vi "Lab Panel V5.11.vi"() -> ()   [LabVIEW 2013] (continued)
                        }
                        n855 = Bundle(cluster=w1527, "STATUS"="STOP") -> (w1525:T4)  [unwired: 2 in]
                        n856 = local write "DISP LAB04-1"(w1525) -> ()
                      }
                    }
                  }
                  frame True {
                    n857 = local read "SIG LAB04-1"() -> (w1534:T2)
                    n858 = stacked-sequence {
                      seq-local: [w1545 _] -> [_ w1549]
                      tunnel: w1543 -> [_ w1559]
                      tunnel: w1542 -> [_ w1558]
                      tunnel: w1541 -> [_ w1557]
                      tunnel: w1540 -> [_ w1556]
                      tunnel: w1539 -> [_ w1555]
                      tunnel: [_ w1554] -> w1538
                      tunnel: w1537 -> [_ w1553]
                      tunnel: w1536 -> [_ w1552]
                      tunnel: w1535 -> [_ w1551]
                      tunnel: w1534 -> [w1544 w1550]
                      tunnel: w1533 -> [_ w1548]
                      frame #0 {
                        n859 = Unbundle(w1544) -> ("AMPS"=w1547:dbl)  [unwired: 4 out]
                        n860 = call "Check For Amps on v1.vi"("ID"="LAB04-1", "amps"=w1547) -> ("amps"=w1545:bool)  [unwired: 9 in]
                      }
                      frame #1 {
                        n861 = case shown="True" w1549 {
                          tunnel: w1559 -> [_ w1572]
                          tunnel: w1558 -> [_ w1571]
                          tunnel: w1557 -> [_ w1570]
                          tunnel: w1556 -> [_ w1569]
                          tunnel: w1555 -> [_ w1568]
                          tunnel: [errorcluster {"status"=FALSE, "code"=0, "source"=""} ("error out") w1567] -> w1554
                          tunnel: w1553 -> [_ w1566]
                          tunnel: w1552 -> [_ w1565]
                          tunnel: w1551 -> [_ w1564]
                          tunnel: w1550 -> [_ w1563]
                          tunnel: w1548 -> [_ w1562]
                          frame False {
                            w1560 = FALSE
                            n862 = local write "RUN LAB04-1"(w1560) -> ()
                            n863 = local write "run lab04-1"(w1560) -> ()
                          }
                          frame True {
                            n864 = stacked-sequence {
                              seq-local: [w1573 _ _ _ _] -> [_ w1597 _ _ _]
                              tunnel: w1572 -> [w1578 _ _ _ _]
                              tunnel: w1571 -> [w1574 _ _ _ _]
                              tunnel: w1570 -> [w1588 _ _ _ _]
                              tunnel: w1569 -> [w1581 _ _ _ _]
                              tunnel: w1568 -> [w1576 _ _ _ _]
                              tunnel: [_ w1592 _ _ _] -> w1567
                              tunnel: w1566 -> [_ _ _ w1618 _]
                              tunnel: w1565 -> [_ _ _ w1617 _]
                              tunnel: w1564 -> [_ _ _ w1616 _]
                              tunnel: w1563 -> [_ _ _ _ _]
                              tunnel: w1562 -> [_ _ _ _ w1632]
                              frame #0 {
                                w1575 = "\\"
                                n865 = local read "SET LAB04-1"() -> (w1583:T5)
                                n866 = case shown="\"CYCLE TEST\"" w1588 {
                                tunnel: ["L04-1-CHART TEST-" "L04-1-CYCLE TEST-" "L04-1-T-RISE TEST-"] -> w1584
                                frame "CHART TEST", Default {
                                }
                                frame "CYCLE TEST" {
                                }
                                frame "T-RISE TEST" {
                                }
                                }
                                n867 = Unbundle(w1583) -> ("DESCRIPTION"=w1582:string)  [unwired: 4 out]
                                n868 = Concatenate Strings(w1578, "\\", w1576, w1575, w1574, w1575) -> (w1585:string)
                                n869 = String To Path(string=w1585) -> (path=w1587:path)
                                n870 = Concatenate Strings(w1585, w1584, w1582, "-", w1581, ".tdms") -> (w1573:string)
                                n871 = Create Folder(path (use dialog)=w1587) -> (error out=w1586:errorcluster)  [unwired: 2 in, 2 out]
                                n872 = global write "Global 1.vi" "LAB04-1 FILE"(w1573) -> ()
                                n873 = call <vilib>:"Clear Errors.vi"("error in (no error)"=w1586) -> ()  [unwired: 6 in, 1 out]
                              }
                              frame #1 {
                                (unwired) FALSE
                                n874 = String To Path(string=w1597) -> (path=w1593:path)
                                n875 = TDMS Open(6:FALSE, 10:T20."create or replace" ("operation (0:open)"), 11:w1593) -> (0:w1592:errorcluster, 3:→"TDMS LAB04-1":refnum<k34>)  [unwired: 4 in]
                              }
                              frame #2 {
                                n876 = local read "SET LAB04-1"() -> (w1603:T5)
                                n877 = local read "TDMS LAB04-1"() -> (w1614:refnum<k34>)
                                n878 = Build Array("Testers Name", "Description", "Set Test Cycles", "T-Rise minutes", "T-Rise Deg C") -> (w1604:string[])
                                n879 = Unbundle(w1603) -> ("NAME"=w1602:string, "DESCRIPTION"=w1601:string, "CYCLES"=w1600:dbl, "T-RISE mins"=w1599:dbl, "T-RISE deg C"=w1598:dbl)
                                n880 = Number To Decimal String(number=w1600) -> (decimal integer string=w1613:string)  [unwired: 1 in]
                                n881 = Number To Decimal String(number=w1599) -> (decimal integer string=w1612:string)  [unwired: 1 in]
                                n882 = Number To Decimal String(number=w1598) -> (decimal integer string=w1611:string)  [unwired: 1 in]
                                n883 = Build Array(w1602, w1601, w1613, w1612, w1611) -> (w1610:string[])
                                n884 = TDMS Set Properties(5:w1610, 7:w1604, 11:w1614) -> ()  [unwired: 3 in, 4 out]
                              }
                              frame #3 {
                                n885 = local read "DISP LAB04-1"() -> (w1619:T4)
                                n886 = Concatenate Strings("LAB04-1  ", w1618) -> (w1620:string)
                                n887 = Two Button Dialog(message=w1620, 1:w1616, 2:w1617) -> (T button?=w1622:bool)
                                n888 = case shown="True" w1622 {
                                tunnel: w1619 -> [w1629 w1630]
                                tunnel: [w1629 w1630] -> w1626
                                tunnel: [w1628 w1631] -> w1625
                                tunnel: [w1627 w1631] -> w1624
                                frame False {
                                n889 = Unbundle(w1629) -> ("CYCLE"=w1628:dbl, "MINS"=w1627:dbl)  [unwired: 1 out]
                                }
                                frame True {
                                w1631 = 0.0
                                }
                                }
                                n890 = Bundle(cluster=w1626, "CYCLE"=w1625, "MINS"=w1624, "STATUS"="RUN") -> (w1615:T4)
                                n891 = local write "DISP LAB04-1"(w1615) -> ()
                              }
                              frame #4 {
                                n892 = local read "TEMP START LAB04-1"() -> (w1634:cluster{"TL":dbl, "TN":dbl})
                                n893 = Bundle(cluster=w1634, "TL"=w1632, "TN"=w1632) -> (w1633:cluster{"TL":dbl, "TN":dbl})
                                n894 = local write "TEMP START LAB04-1"(w1633) -> ()
                              }
                            }
                          }
                        }
                      }
                    }
                  }
                }
              }
              event "RUN LAB04-2": Value Change {
                n895 = event-data() -> ("NewVal"=w1639:bool)  [unwired: 1 in, 5 out]
                n896 = local write "run lab04-2"(w1639) -> ()
                n897 = case shown="True" w1639 {
                  tunnel: w1645 -> [_ w1683]
                  tunnel: w1644 -> [_ w1682]
                  tunnel: w1642 -> [w1647 w1681]
                  tunnel: w1643 -> [_ w1680]
                  tunnel: w1641 -> [_ w1679]
                  tunnel: [w1646 w1678] -> w1640
                  tunnel: w1638 -> [_ w1677]
                  tunnel: w1637 -> [_ w1676]
                  tunnel: w1636 -> [_ w1675]
                  tunnel: w1635 -> [_ w1673]
                  frame False {
                    # "stop test"
                    n898 = stacked-sequence {
                      tunnel: w1647 -> [w1656 _]
                      tunnel: [w1648 _] -> w1646
                      frame #0 {
                        n899 = local read "DISP LAB04-2"() -> (w1655:T4)
                        n900 = Unbundle(w1655) -> ("CYCLE"=w1653:dbl, "MINS"=w1654:dbl)  [unwired: 1 out]
                        n901 = case shown="\"CYCLE TEST\"" w1656 {
                          tunnel: w1654 -> [_ _ w1663]
                          tunnel: w1653 -> [w1661 w1662 _]
                          tunnel: [w1661 w1662 w1663] -> w1652
                          frame "CHART TEST", Default {
                          }
                          frame "CYCLE TEST" {
                          }
                          frame "T-RISE TEST" {
                          }
                        }
                        n902 = local read "TDMS LAB04-2"() -> (w1660:refnum<k34>)
                        n903 = Build Array("STOPPED") -> (w1657:string[])
                        n904 = Build Array(w1652) -> (w1651:dbl[])
                        n905 = TDMS Write(0:w1660, 5:"TEST RESULT", 7:w1657, 9:w1651) -> (4:w1649:refnum<k34>, 15:w1650:errorcluster)  [unwired: 2 in, 2 out]
                        n906 = TDMS Close(8:w1650, 11:w1649) -> (0:w1648:errorcluster)  [unwired: 1 out]
                      }
                      frame #1 {
                        n907 = local read "DISP LAB04-2"() -> (w1667:T4)
                        n908 = stacked-sequence {
                          tunnel: "LAB04-2" -> [w1669 w1671]
                          frame #0 {
                            n909 = call "sub vi - defrag tdms v1.vi"("panel id"=w1669) -> ("error out"=w1668:errorcluster)  [unwired: 10 in]
                            n910 = local write "data file error"(w1668) -> ()
                          }
                          frame #1 {
                            n911 = call "Save data file (stop) v3.vi"("panel id"=w1671) -> ("network file save error"=w1670:errorcluster)  [unwired: 9 in, 1 out]
                            n912 = local write "RESULT LAB04-2"(FALSE) -> ()
                            n913 = local write "data file error"(w1670) -> ()
                          }
                        }
                        n914 = Bundle(cluster=w1667, "STATUS"="STOP") -> (w1665:T4)  [unwired: 2 in]
                        n915 = local write "DISP LAB04-2"(w1665) -> ()
                      }
                    }
                  }
                  frame True {
                    n916 = local read "SIG LAB04-2"() -> (w1674:T2)
                    n917 = stacked-sequence {
                      seq-local: [w1685 _] -> [_ w1689]
                      tunnel: w1683 -> [_ w1699]
                      tunnel: w1682 -> [_ w1698]
                      tunnel: w1681 -> [_ w1697]
                      tunnel: w1680 -> [_ w1696]
                      tunnel: w1679 -> [_ w1695]
                      tunnel: [_ w1694] -> w1678
                      tunnel: w1677 -> [_ w1693]
                      tunnel: w1676 -> [_ w1692]
                      tunnel: w1675 -> [_ w1691]
                      tunnel: w1674 -> [w1684 w1690]
                      tunnel: w1673 -> [_ w1688]
                      frame #0 {
                        n918 = Unbundle(w1684) -> ("AMPS"=w1687:dbl)  [unwired: 4 out]
                        n919 = call "Check For Amps on v1.vi"("ID"="LAB04-2", "amps"=w1687) -> ("amps"=w1685:bool)  [unwired: 9 in]
                      }
                      frame #1 {
                        n920 = case shown="True" w1689 {
                          tunnel: w1699 -> [_ w1712]
                          tunnel: w1698 -> [_ w1711]
                          tunnel: w1697 -> [_ w1710]
                          tunnel: w1696 -> [_ w1709]
                          tunnel: w1695 -> [_ w1708]
                          tunnel: [errorcluster {"status"=FALSE, "code"=0, "source"=""} ("error out") w1707] -> w1694
                          tunnel: w1693 -> [_ w1706]
                          tunnel: w1692 -> [_ w1705]
                          tunnel: w1691 -> [_ w1704]
                          tunnel: w1690 -> [_ w1703]
                          tunnel: w1688 -> [_ w1702]
                          frame False {
                            w1700 = FALSE
                            n921 = local write "RUN LAB04-2"(w1700) -> ()
                            n922 = local write "run lab04-2"(w1700) -> ()
                          }
                          frame True {
                            n923 = stacked-sequence {
                              seq-local: [w1713 _ _ _ _] -> [_ w1737 _ _ _]
                              tunnel: w1712 -> [w1718 _ _ _ _]
                              tunnel: w1711 -> [w1714 _ _ _ _]
                              tunnel: w1710 -> [w1728 _ _ _ _]
                              tunnel: w1709 -> [w1721 _ _ _ _]
                              tunnel: w1708 -> [w1716 _ _ _ _]
                              tunnel: [_ w1732 _ _ _] -> w1707
                              tunnel: w1706 -> [_ _ _ w1758 _]
                              tunnel: w1705 -> [_ _ _ w1757 _]
                              tunnel: w1704 -> [_ _ _ w1756 _]
                              tunnel: w1703 -> [_ _ _ _ _]
                              tunnel: w1702 -> [_ _ _ _ w1772]
                              frame #0 {
                                w1715 = "\\"
                                n924 = local read "SET LAB04-2"() -> (w1723:T5)
                                n925 = case shown="\"CHART TEST\", Default" w1728 {
                                tunnel: ["L04-2-CHART TEST-" "L04-2-CYCLE TEST-" "L04-2-T-RISE TEST-"] -> w1724
                                frame "CHART TEST", Default {
                                }
                                frame "CYCLE TEST" {
                                }
                                frame "T-RISE TEST" {
                                }
                                }
                                n926 = Unbundle(w1723) -> ("DESCRIPTION"=w1722:string)  [unwired: 4 out]
                                n927 = Concatenate Strings(w1718, "\\", w1716, w1715, w1714, w1715) -> (w1725:string)
                                n928 = String To Path(string=w1725) -> (path=w1727:path)
                                n929 = Concatenate Strings(w1725, w1724, w1722, "-", w1721, ".tdms") -> (w1713:string)
                                n930 = Create Folder(path (use dialog)=w1727) -> (error out=w1726:errorcluster)  [unwired: 2 in, 2 out]
                                n931 = global write "Global 1.vi" "LAB04-2 FILE"(w1713) -> ()
                                n932 = call <vilib>:"Clear Errors.vi"("error in (no error)"=w1726) -> ()  [unwired: 6 in, 1 out]
                              }
                              frame #1 {
                                (unwired) FALSE
                                n933 = String To Path(string=w1737) -> (path=w1733:path)
                                n934 = TDMS Open(6:FALSE, 10:T20."create or replace" ("operation (0:open)"), 11:w1733) -> (0:w1732:errorcluster, 3:→"TDMS LAB04-2":refnum<k34>)  [unwired: 4 in]
                              }
                              frame #2 {
                                n935 = local read "SET LAB04-2"() -> (w1743:T5)
                                n936 = local read "TDMS LAB04-2"() -> (w1754:refnum<k34>)
                                n937 = Build Array("Testers Name", "Description", "Set Test Cycles", "T-Rise minutes", "T-Rise Deg C") -> (w1744:string[])
                                n938 = Unbundle(w1743) -> ("NAME"=w1742:string, "DESCRIPTION"=w1741:string, "CYCLES"=w1740:dbl, "T-RISE mins"=w1739:dbl, "T-RISE deg C"=w1738:dbl)
                                n939 = Number To Decimal String(number=w1740) -> (decimal integer string=w1753:string)  [unwired: 1 in]
                                n940 = Number To Decimal String(number=w1739) -> (decimal integer string=w1752:string)  [unwired: 1 in]
                                n941 = Number To Decimal String(number=w1738) -> (decimal integer string=w1751:string)  [unwired: 1 in]
                                n942 = Build Array(w1742, w1741, w1753, w1752, w1751) -> (w1750:string[])
                                n943 = TDMS Set Properties(5:w1750, 7:w1744, 11:w1754) -> ()  [unwired: 3 in, 4 out]
                              }
                              frame #3 {
                                n944 = local read "DISP LAB04-2"() -> (w1759:T4)
                                n945 = Concatenate Strings("LAB04-2 ", w1758) -> (w1760:string)
                                n946 = Two Button Dialog(message=w1760, 1:w1756, 2:w1757) -> (T button?=w1762:bool)
                                n947 = case shown="True" w1762 {
                                tunnel: w1759 -> [w1769 w1770]
                                tunnel: [w1769 w1770] -> w1766
                                tunnel: [w1768 w1771] -> w1765
                                tunnel: [w1767 w1771] -> w1764
                                frame False {
                                n948 = Unbundle(w1769) -> ("CYCLE"=w1768:dbl, "MINS"=w1767:dbl)  [unwired: 1 out]
                                }
                                frame True {
                                w1771 = 0.0
                                }
                                }
                                n949 = Bundle(cluster=w1766, "CYCLE"=w1765, "MINS"=w1764, "STATUS"="RUN") -> (w1755:T4)
                                n950 = local write "DISP LAB04-2"(w1755) -> ()
                              }
                              frame #4 {
                                n951 = local read "TEMP START LAB04-2"() -> (w1774:cluster{"TL":dbl, "TN":dbl})
                                n952 = Bundle(cluster=w1774, "TL"=w1772, "TN"=w1772) -> (w1773:cluster{"TL":dbl, "TN":dbl})
                                n953 = local write "TEMP START LAB04-2"(w1773) -> ()
                              }
                            }
                          }
                        }
                      }
                    }
                  }
                }
              }
              event "RUN LAB05-1": Value Change {
                n954 = event-data() -> ("NewVal"=w1779:bool)  [unwired: 1 in, 5 out]
                n955 = local write "run lab05-1"(w1779) -> ()
                n956 = case shown="True" w1779 {
                  tunnel: w1785 -> [_ w1823]
                  tunnel: w1784 -> [_ w1822]
                  tunnel: w1782 -> [w1787 w1821]
                  tunnel: w1783 -> [_ w1820]
                  tunnel: w1781 -> [_ w1819]
                  tunnel: [w1786 w1818] -> w1780
                  tunnel: w1778 -> [_ w1817]
                  tunnel: w1777 -> [_ w1816]
                  tunnel: w1776 -> [_ w1815]
                  tunnel: w1775 -> [_ w1813]
                  frame False {
                    # "stop test"
                    n957 = stacked-sequence {
                      tunnel: w1787 -> [w1796 _]
                      tunnel: [w1788 _] -> w1786
                      frame #0 {
                        n958 = local read "DISP LAB05-1"() -> (w1795:T4)
                        n959 = Unbundle(w1795) -> ("CYCLE"=w1793:dbl, "MINS"=w1794:dbl)  [unwired: 1 out]
                        n960 = case shown="\"CYCLE TEST\"" w1796 {
                          tunnel: w1794 -> [_ _ w1803]
                          tunnel: w1793 -> [w1801 w1802 _]
                          tunnel: [w1801 w1802 w1803] -> w1792
                          frame "CHART TEST", Default {
                          }
                          frame "CYCLE TEST" {
                          }
                          frame "T-RISE TEST" {
                          }
                        }
                        n961 = local read "TDMS LAB05-1"() -> (w1800:refnum<k34>)
                        n962 = Build Array("STOPPED") -> (w1797:string[])
                        n963 = Build Array(w1792) -> (w1791:dbl[])
                        n964 = TDMS Write(0:w1800, 5:"TEST RESULT", 7:w1797, 9:w1791) -> (4:w1789:refnum<k34>, 15:w1790:errorcluster)  [unwired: 2 in, 2 out]
                        n965 = TDMS Close(8:w1790, 11:w1789) -> (0:w1788:errorcluster)  [unwired: 1 out]
                      }
                      frame #1 {
                        n966 = local read "DISP LAB05-1"() -> (w1807:T4)
                        n967 = stacked-sequence {
                          tunnel: "LAB05-1" -> [w1809 w1811]
                          frame #0 {
                            n968 = call "sub vi - defrag tdms v1.vi"("panel id"=w1809) -> ("error out"=w1808:errorcluster)  [unwired: 10 in]
                            n969 = local write "data file error"(w1808) -> ()
                          }
                          frame #1 {
                            n970 = call "Save data file (stop) v3.vi"("panel id"=w1811) -> ("network file save error"=w1810:errorcluster)  [unwired: 9 in, 1 out]
                            n971 = local write "RESULT LAB05-1"(FALSE) -> ()
                            n972 = local write "data file error"(w1810) -> ()
                          }
                        }
                        n973 = Bundle(cluster=w1807, "STATUS"="STOP") -> (w1805:T4)  [unwired: 2 in]
                        n974 = local write "DISP LAB05-1"(w1805) -> ()
                      }
                    }
                  }
                  frame True {
                    n975 = local read "SIG LAB05-1"() -> (w1814:T2)
                    n976 = stacked-sequence {
                      seq-local: [w1825 _] -> [_ w1829]
                      tunnel: w1823 -> [_ w1839]
                      tunnel: w1822 -> [_ w1838]
                      tunnel: w1821 -> [_ w1837]
                      tunnel: w1820 -> [_ w1836]
                      tunnel: w1819 -> [_ w1835]
                      tunnel: [_ w1834] -> w1818
                      tunnel: w1817 -> [_ w1833]
                      tunnel: w1816 -> [_ w1832]
                      tunnel: w1815 -> [_ w1831]
                      tunnel: w1814 -> [w1824 w1830]
                      tunnel: w1813 -> [_ w1828]
                      frame #0 {
                        n977 = Unbundle(w1824) -> ("AMPS"=w1827:dbl)  [unwired: 4 out]
                        n978 = call "Check For Amps on v1.vi"("ID"="LAB05-1", "amps"=w1827) -> ("amps"=w1825:bool)  [unwired: 9 in]
                      }
                      frame #1 {
                        n979 = case shown="True" w1829 {
                          tunnel: w1839 -> [_ w1852]
                          tunnel: w1838 -> [_ w1851]
                          tunnel: w1837 -> [_ w1850]
                          tunnel: w1836 -> [_ w1849]
                          tunnel: w1835 -> [_ w1848]
                          tunnel: [errorcluster {"status"=FALSE, "code"=0, "source"=""} ("error out") w1847] -> w1834
                          tunnel: w1833 -> [_ w1846]
                          tunnel: w1832 -> [_ w1845]
                          tunnel: w1831 -> [_ w1844]
                          tunnel: w1830 -> [_ w1843]
                          tunnel: w1828 -> [_ w1842]
                          frame False {
                            w1840 = FALSE
                            n980 = local write "RUN LAB05-1"(w1840) -> ()
                            n981 = local write "run lab05-1"(w1840) -> ()
                          }
                          frame True {
                            n982 = stacked-sequence {
                              seq-local: [w1853 _ _ _ _] -> [_ w1877 _ _ _]
                              tunnel: w1852 -> [w1858 _ _ _ _]
                              tunnel: w1851 -> [w1854 _ _ _ _]
                              tunnel: w1850 -> [w1868 _ _ _ _]
                              tunnel: w1849 -> [w1861 _ _ _ _]
                              tunnel: w1848 -> [w1856 _ _ _ _]
                              tunnel: [_ w1872 _ _ _] -> w1847
                              tunnel: w1846 -> [_ _ _ w1897 _]
                              tunnel: w1845 -> [_ _ _ w1896 _]
                              tunnel: w1844 -> [_ _ _ w1895 _]
                              tunnel: w1843 -> [_ _ _ _ _]
                              tunnel: w1842 -> [_ _ _ _ w1912]
                              frame #0 {
                                w1855 = "\\"
                                n983 = local read "SET LAB05-1"() -> (w1863:T5)
                                n984 = case shown="\"CYCLE TEST\"" w1868 {
                                tunnel: ["L05-1-CHART TEST-" "L05-1-CYCLE TEST-" "L05-1-T-RISE TEST-"] -> w1864
                                frame "CHART TEST", Default {
                                }
                                frame "CYCLE TEST" {
                                }
                                frame "T-RISE TEST" {
                                }
                                }
                                n985 = Unbundle(w1863) -> ("DESCRIPTION"=w1862:string)  [unwired: 4 out]
                                n986 = Concatenate Strings(w1858, "\\", w1856, w1855, w1854, w1855) -> (w1865:string)
                                n987 = String To Path(string=w1865) -> (path=w1867:path)
                                n988 = Concatenate Strings(w1865, w1864, w1862, "-", w1861, ".tdms") -> (w1853:string)
                                n989 = Create Folder(path (use dialog)=w1867) -> (error out=w1866:errorcluster)  [unwired: 2 in, 2 out]
                                n990 = global write "Global 1.vi" "LAB05-1 FILE"(w1853) -> ()
                                n991 = call <vilib>:"Clear Errors.vi"("error in (no error)"=w1866) -> ()  [unwired: 6 in, 1 out]
                              }
                              frame #1 {
                                (unwired) FALSE
                                n992 = String To Path(string=w1877) -> (path=w1873:path)
                                n993 = TDMS Open(6:FALSE, 10:T20."create or replace" ("operation (0:open)"), 11:w1873) -> (0:w1872:errorcluster, 3:→"TDMS LAB05-1":refnum<k34>)  [unwired: 4 in]
                              }
                              frame #2 {
                                n994 = local read "SET LAB05-1"() -> (w1883:T5)
                                n995 = local read "TDMS LAB05-1"() -> (w1894:refnum<k34>)
                                n996 = Build Array("Testers Name", "Description", "Set Test Cycles", "T-Rise minutes", "T-Rise Deg C") -> (w1884:string[])
                                n997 = Unbundle(w1883) -> ("NAME"=w1882:string, "DESCRIPTION"=w1881:string, "CYCLES"=w1880:dbl, "T-RISE mins"=w1879:dbl, "T-RISE deg C"=w1878:dbl)
                                n998 = Number To Decimal String(number=w1880) -> (decimal integer string=w1893:string)  [unwired: 1 in]
                                n999 = Number To Decimal String(number=w1879) -> (decimal integer string=w1892:string)  [unwired: 1 in]
                                n1000 = Number To Decimal String(number=w1878) -> (decimal integer string=w1891:string)  [unwired: 1 in]
                                n1001 = Build Array(w1882, w1881, w1893, w1892, w1891) -> (w1890:string[])
                                n1002 = TDMS Set Properties(5:w1890, 7:w1884, 11:w1894) -> ()  [unwired: 3 in, 4 out]
                              }
                              frame #3 {
                                n1003 = local read "DISP LAB05-1"() -> (w1899:T4)
                                n1004 = Concatenate Strings("LAB05-1  ", w1897) -> (w1900:string)
                                n1005 = Two Button Dialog(message=w1900, 1:w1895, 2:w1896) -> (T button?=w1902:bool)
                                n1006 = case shown="True" w1902 {
                                tunnel: w1899 -> [w1909 w1910]
                                tunnel: [w1909 w1910] -> w1906
                                tunnel: [w1908 w1911] -> w1905
                                tunnel: [w1907 w1911] -> w1904
                                frame False {
                                n1007 = Unbundle(w1909) -> ("CYCLE"=w1908:dbl, "MINS"=w1907:dbl)  [unwired: 1 out]
                                }
                                frame True {
                                w1911 = 0.0
                                }
                                }
                                n1008 = Bundle(cluster=w1906, "CYCLE"=w1905, "MINS"=w1904, "STATUS"="RUN") -> (w1898:T4)
                                n1009 = local write "DISP LAB05-1"(w1898) -> ()
                              }
                              frame #4 {
                                n1010 = local read "TEMP START LAB05-1"() -> (w1914:cluster{"TL":dbl, "TN":dbl})
                                n1011 = Bundle(cluster=w1914, "TL"=w1912, "TN"=w1912) -> (w1913:cluster{"TL":dbl, "TN":dbl})
                                n1012 = local write "TEMP START LAB05-1"(w1913) -> ()
                              }
                            }
                          }
                        }
                      }
                    }
                  }
                }
              }
              event "RUN LAB05-2": Value Change {
                n1013 = event-data() -> ("NewVal"=w1920:bool)  [unwired: 1 in, 5 out]
                n1014 = local read "SIG LAB05-2"() -> (w1916:T2)
                n1015 = case shown="True" w1920 {
                  tunnel: w1926 -> [_ w1964]
                  tunnel: w1925 -> [_ w1963]
                  tunnel: w1923 -> [w1928 w1962]
                  tunnel: w1924 -> [_ w1961]
                  tunnel: w1922 -> [_ w1960]
                  tunnel: [w1927 w1959] -> w1921
                  tunnel: w1919 -> [_ w1958]
                  tunnel: w1918 -> [_ w1957]
                  tunnel: w1917 -> [_ w1956]
                  tunnel: w1916 -> [_ w1955]
                  tunnel: w1915 -> [_ w1954]
                  frame False {
                    # "stop test"
                    n1016 = stacked-sequence {
                      tunnel: w1928 -> [w1937 _]
                      tunnel: [w1929 _] -> w1927
                      frame #0 {
                        n1017 = local read "DISP LAB05-2"() -> (w1936:T4)
                        n1018 = Unbundle(w1936) -> ("CYCLE"=w1934:dbl, "MINS"=w1935:dbl)  [unwired: 1 out]
                        n1019 = case shown="\"CYCLE TEST\"" w1937 {
                          tunnel: w1935 -> [_ _ w1944]
                          tunnel: w1934 -> [w1942 w1943 _]
                          tunnel: [w1942 w1943 w1944] -> w1933
                          frame "CHART TEST", Default {
                          }
                          frame "CYCLE TEST" {
                          }
                          frame "T-RISE TEST" {
                          }
                        }
                        n1020 = local read "TDMS LAB05-2"() -> (w1941:refnum<k34>)
                        n1021 = Build Array("STOPPED") -> (w1938:string[])
                        n1022 = Build Array(w1933) -> (w1932:dbl[])
                        n1023 = TDMS Write(0:w1941, 5:"TEST RESULT", 7:w1938, 9:w1932) -> (4:w1930:refnum<k34>, 15:w1931:errorcluster)  [unwired: 2 in, 2 out]
                        n1024 = TDMS Close(8:w1931, 11:w1930) -> (0:w1929:errorcluster)  [unwired: 1 out]
                      }
                      frame #1 {
                        n1025 = local read "DISP LAB05-2"() -> (w1948:T4)
                        n1026 = stacked-sequence {
                          tunnel: "LAB05-2" -> [w1950 w1952]
                          frame #0 {
                            n1027 = call "sub vi - defrag tdms v1.vi"("panel id"=w1950) -> ("error out"=w1949:errorcluster)  [unwired: 10 in]
                            n1028 = local write "data file error"(w1949) -> ()
                          }
                          frame #1 {
                            n1029 = local write "RESULT LAB05-2"(FALSE) -> ()
                            n1030 = call "Save data file (stop) v3.vi"("panel id"=w1952) -> ("network file save error"=w1951:errorcluster)  [unwired: 9 in, 1 out]
                            n1031 = local write "data file error"(w1951) -> ()
                          }
                        }
                        n1032 = Bundle(cluster=w1948, "STATUS"="STOP") -> (w1946:T4)  [unwired: 2 in]
                        n1033 = local write "DISP LAB05-2"(w1946) -> ()
                      }
                    }
                  }
                  frame True {
                    n1034 = stacked-sequence {
                      seq-local: [w1966 _] -> [_ w1970]
                      tunnel: w1964 -> [_ w1980]
                      tunnel: w1963 -> [_ w1979]
                      tunnel: w1962 -> [_ w1978]
                      tunnel: w1961 -> [_ w1977]
                      tunnel: w1960 -> [_ w1976]
                      tunnel: [_ w1975] -> w1959
                      tunnel: w1958 -> [_ w1974]
                      tunnel: w1957 -> [_ w1973]
                      tunnel: w1956 -> [_ w1972]
                      tunnel: w1955 -> [w1965 w1971]
                      tunnel: w1954 -> [_ w1969]
                      frame #0 {
                        n1035 = Unbundle(w1965) -> ("AMPS"=w1968:dbl)  [unwired: 4 out]
                        n1036 = call "Check For Amps on v1.vi"("ID"="LAB05-2", "amps"=w1968) -> ("amps"=w1966:bool)  [unwired: 9 in]
                      }
                      frame #1 {
                        n1037 = case shown="True" w1970 {
                          tunnel: w1980 -> [_ w1993]
                          tunnel: w1979 -> [_ w1992]
                          tunnel: w1978 -> [_ w1991]
                          tunnel: w1977 -> [_ w1990]
                          tunnel: w1976 -> [_ w1989]
                          tunnel: [errorcluster {"status"=FALSE, "code"=0, "source"=""} ("error out") w1988] -> w1975
                          tunnel: w1974 -> [_ w1987]
                          tunnel: w1973 -> [_ w1986]
                          tunnel: w1972 -> [_ w1985]
                          tunnel: w1971 -> [_ w1984]
                          tunnel: w1969 -> [_ w1983]
                          frame False {
                            w1981 = FALSE
                            n1038 = local write "RUN LAB05-2"(w1981) -> ()
                            n1039 = local write "run lab05-2"(w1981) -> ()
                          }
                          frame True {
                            n1040 = stacked-sequence {
                              seq-local: [w1994 _ _ _ _] -> [_ w2018 _ _ _]
                              tunnel: w1993 -> [w1999 _ _ _ _]
                              tunnel: w1992 -> [w1995 _ _ _ _]
                              tunnel: w1991 -> [w2009 _ _ _ _]
                              tunnel: w1990 -> [w2002 _ _ _ _]
                              tunnel: w1989 -> [w1997 _ _ _ _]
                              tunnel: [_ w2013 _ _ _] -> w1988
                              tunnel: w1987 -> [_ _ _ w2038 _]
                              tunnel: w1986 -> [_ _ _ w2037 _]
                              tunnel: w1985 -> [_ _ _ w2036 _]
                              tunnel: w1984 -> [_ _ _ _ _]
                              tunnel: w1983 -> [_ _ _ _ w2053]
                              frame #0 {
                                w1996 = "\\"
                                n1041 = local read "SET LAB05-2"() -> (w2004:T5)
                                n1042 = case shown="\"CYCLE TEST\"" w2009 {
                                tunnel: ["L05-2-CHART TEST-" "L05-2-CYCLE TEST-" "L05-2-T-RISE TEST-"] -> w2005
                                frame "CHART TEST", Default {
                                }
                                frame "CYCLE TEST" {
                                }
                                frame "T-RISE TEST" {
                                }
                                }
                                n1043 = Unbundle(w2004) -> ("DESCRIPTION"=w2003:string)  [unwired: 4 out]
                                n1044 = Concatenate Strings(w1999, "\\", w1997, w1996, w1995, w1996) -> (w2006:string)
                                n1045 = String To Path(string=w2006) -> (path=w2008:path)
                                n1046 = Concatenate Strings(w2006, w2005, w2003, "-", w2002, ".tdms") -> (w1994:string)
                                n1047 = Create Folder(path (use dialog)=w2008) -> (error out=w2007:errorcluster)  [unwired: 2 in, 2 out]
                                n1048 = global write "Global 1.vi" "LAB05-2 FILE"(w1994) -> ()
                                n1049 = call <vilib>:"Clear Errors.vi"("error in (no error)"=w2007) -> ()  [unwired: 6 in, 1 out]
                              }
                              frame #1 {
                                (unwired) FALSE
                                n1050 = String To Path(string=w2018) -> (path=w2014:path)
                                n1051 = TDMS Open(6:FALSE, 10:T20."create or replace" ("operation (0:open)"), 11:w2014) -> (0:w2013:errorcluster, 3:→"TDMS LAB05-2":refnum<k34>)  [unwired: 4 in]
                              }
                              frame #2 {
                                n1052 = local read "SET LAB05-2"() -> (w2024:T5)
                                n1053 = local read "TDMS LAB05-2"() -> (w2035:refnum<k34>)
                                n1054 = Build Array("Testers Name", "Description", "Set Test Cycles", "T-Rise minutes", "T-Rise Deg C") -> (w2025:string[])
                                n1055 = Unbundle(w2024) -> ("NAME"=w2023:string, "DESCRIPTION"=w2022:string, "CYCLES"=w2021:dbl, "T-RISE mins"=w2020:dbl, "T-RISE deg C"=w2019:dbl)
                                n1056 = Number To Decimal String(number=w2021) -> (decimal integer string=w2034:string)  [unwired: 1 in]
                                n1057 = Number To Decimal String(number=w2020) -> (decimal integer string=w2033:string)  [unwired: 1 in]
                                n1058 = Number To Decimal String(number=w2019) -> (decimal integer string=w2032:string)  [unwired: 1 in]
                                n1059 = Build Array(w2023, w2022, w2034, w2033, w2032) -> (w2031:string[])
                                n1060 = TDMS Set Properties(5:w2031, 7:w2025, 11:w2035) -> ()  [unwired: 3 in, 4 out]
                              }
                              frame #3 {
                                n1061 = local read "DISP LAB05-2"() -> (w2040:T4)
                                n1062 = Concatenate Strings("LAB05-2  ", w2038) -> (w2041:string)
                                n1063 = Two Button Dialog(message=w2041, 1:w2036, 2:w2037) -> (T button?=w2043:bool)
                                n1064 = case shown="True" w2043 {
                                tunnel: w2040 -> [w2050 w2051]
                                tunnel: [w2050 w2051] -> w2047
                                tunnel: [w2049 w2052] -> w2046
                                tunnel: [w2048 w2052] -> w2045
                                frame False {
                                n1065 = Unbundle(w2050) -> ("CYCLE"=w2049:dbl, "MINS"=w2048:dbl)  [unwired: 1 out]
                                }
                                frame True {
                                w2052 = 0.0
                                }
                                }
                                n1066 = Bundle(cluster=w2047, "CYCLE"=w2046, "MINS"=w2045, "STATUS"="RUN") -> (w2039:T4)
                                n1067 = local write "DISP LAB05-2"(w2039) -> ()
                              }
                              frame #4 {
                                n1068 = local read "TEMP START LAB05-2"() -> (w2055:cluster{"TL":dbl, "TN":dbl})
                                n1069 = Bundle(cluster=w2055, "TL"=w2053, "TN"=w2053) -> (w2054:cluster{"TL":dbl, "TN":dbl})
                                n1070 = local write "TEMP START LAB05-2"(w2054) -> ()
                              }
                            }
                          }
                        }
                      }
                    }
                  }
                }
                n1071 = local write "run lab05-2"(w1920) -> ()
              }
            }
            n1072 = local write "data file error"(w624) -> ()
          }
          frame #4 {
            # "check if test cycles reached for cycle tests, if so then test pass"
            n1073 = stacked-sequence {
              tunnel: w2075 -> [_ _ _ _ _ _ _ _ _ _]
              tunnel: w2074 -> [_ _ _ _ _ _ _ _ _ _]
              tunnel: w2073 -> [_ _ _ _ _ _ _ _ _ _]
              tunnel: w2072 -> [_ _ _ _ _ _ _ _ _ _]
              tunnel: w2071 -> [_ _ _ _ _ _ _ _ _ _]
              tunnel: w2070 -> [_ _ _ _ _ _ _ _ _ _]
              tunnel: w2069 -> [_ _ _ _ _ _ _ _ _ _]
              tunnel: w2068 -> [_ _ _ _ _ _ _ _ _ _]
              tunnel: w2067 -> [_ _ _ _ _ _ _ _ _ _]
              tunnel: w2066 -> [_ _ _ _ _ _ _ _ _ _]
              tunnel: w2065 -> [w2081 _ _ _ _ _ _ _ _ _]
              tunnel: w2064 -> [_ w2116 _ _ _ _ _ _ _ _]
              tunnel: w2063 -> [_ _ w2156 _ _ _ _ _ _ _]
              tunnel: w2062 -> [_ _ _ w2196 _ _ _ _ _ _]
              tunnel: w2061 -> [_ _ _ _ w2236 _ _ _ _ _]
              tunnel: w2060 -> [_ _ _ _ _ w2276 _ _ _ _]
              tunnel: w2059 -> [_ _ _ _ _ _ w2316 _ _ _]
              tunnel: w2058 -> [_ _ _ _ _ _ _ w2356 _ _]
              tunnel: w2057 -> [_ _ _ _ _ _ _ _ w2396 _]
              tunnel: w2056 -> [_ _ _ _ _ _ _ _ _ w2436]
              frame #0 {
                # "LAB01-1"
                n1074 = Less?(x=w2081, y=2) -> (x < y?=w2079:bool)
                n1075 = local read "DISP LAB01-1"() -> (w2082:T4)
                n1076 = Unbundle(w2082) -> ("STATUS"=w2076:string)  [unwired: 2 out]
                n1077 = Equal?(x=w2076, y="RUN") -> (x = y?=w2078:bool)
                n1078 = And(x=w2078, y=w2079) -> (x .and. y?=w2077:bool)
                n1079 = case shown="True" w2077 {
                  tunnel: w2082 -> [_ w2087]
                  tunnel: w2081 -> [_ w2091]
                  frame False {
                  }
                  frame True {
                    n1080 = local read "SET LAB01-1"() -> (w2093:T5)
                    n1081 = local read "TDMS LAB01-1"() -> (w2086:refnum<k34>)
                    n1082 = Unbundle(w2093) -> ("CYCLES"=w2084:dbl, "T-RISE mins"=w2090:dbl)  [unwired: 3 out]
                    n1083 = case shown="\"CYCLE TEST\"" w2091 {
                      tunnel: w2090 -> [_ _ w2100]
                      tunnel: [w2095 w2097 w2100] -> w2089
                      tunnel: w2084 -> [w2095 w2097 _]
                      tunnel: ["CHART PASS" "CYCLE PASS" "T-RISE PASS"] -> w2088
                      frame "CHART TEST", Default {
                      }
                      frame "CYCLE TEST" {
                      }
                      frame "T-RISE TEST" {
                      }
                    }
                    n1084 = Unbundle(w2087) -> ("CYCLE"=w2092:dbl)  [unwired: 2 out]
                    n1085 = Increment(x=w2084) -> (x+1=w2085:dbl)
                    n1086 = Greater Or Equal?(x=w2092, y=w2085) -> (x >= y?=w2094:bool)
                    n1087 = case shown="True" w2094 {
                      tunnel: w2089 -> [w2104 _]
                      tunnel: w2088 -> [w2103 _]
                      tunnel: w2087 -> [w2102 _]
                      tunnel: w2086 -> [w2101 _]
                      frame True {
                        n1088 = stacked-sequence {
                          tunnel: w2104 -> [w2108 _]
                          tunnel: w2103 -> [w2106 w2112]
                          tunnel: w2102 -> [_ w2115]
                          tunnel: w2101 -> [w2105 _]
                          frame #0 {
                            n1089 = Build Array(w2106) -> (w2109:string[])
                            n1090 = Build Array(w2108) -> (w2107:dbl[])
                            n1091 = TDMS Write(0:w2105, 5:"TEST PASS", 7:w2109, 9:w2107) -> (15:w2111:errorcluster)  [unwired: 2 in, 3 out]
                            n1092 = local write "data file error"(w2111) -> ()
                          }
                          frame #1 {
                            n1093 = Bundle(cluster=w2115, "STATUS"=w2112) -> (w2113:T4)  [unwired: 2 in]
                            n1094 = local write "RESULT LAB01-1"(TRUE) -> ()
                            n1095 = local write "DISP LAB01-1"(w2113) -> ()
                          }
                        }
                      }
                      frame False {
                      }
                    }
                  }
                }
              }
              frame #1 {
                # "LAB01-2"
                n1096 = Less?(x=w2116, y=2) -> (x < y?=w2119:bool)
                n1097 = local read "DISP LAB01-2"() -> (w2121:T4)
                n1098 = Unbundle(w2121) -> ("STATUS"=w2122:string)  [unwired: 2 out]
                n1099 = Equal?(x=w2122, y="RUN") -> (x = y?=w2118:bool)
                n1100 = And(x=w2118, y=w2119) -> (x .and. y?=w2117:bool)
                n1101 = case shown="True" w2117 {
                  tunnel: w2121 -> [_ w2127]
                  tunnel: w2116 -> [_ w2131]
                  frame False {
                  }
                  frame True {
                    n1102 = local read "SET LAB01-2"() -> (w2133:T5)
                    n1103 = local read "TDMS LAB01-2"() -> (w2126:refnum<k34>)
                    n1104 = Unbundle(w2133) -> ("CYCLES"=w2124:dbl, "T-RISE mins"=w2130:dbl)  [unwired: 3 out]
                    n1105 = case shown="\"T-RISE TEST\"" w2131 {
                      tunnel: w2130 -> [_ _ w2140]
                      tunnel: [w2135 w2137 w2140] -> w2129
                      tunnel: w2124 -> [w2135 w2137 _]
                      tunnel: ["CHART PASS" "CYCLE PASS" "T-RISE PASS"] -> w2128
                      frame "CHART TEST", Default {
                      }
                      frame "CYCLE TEST" {
                      }
                      frame "T-RISE TEST" {
                      }
                    }
                    n1106 = Unbundle(w2127) -> ("CYCLE"=w2132:dbl)  [unwired: 2 out]
                    n1107 = Increment(x=w2124) -> (x+1=w2125:dbl)
                    n1108 = Greater Or Equal?(x=w2132, y=w2125) -> (x >= y?=w2134:bool)
                    n1109 = case shown="True" w2134 {
                      tunnel: w2129 -> [w2144 _]
                      tunnel: w2128 -> [w2143 _]
                      tunnel: w2127 -> [w2142 _]
                      tunnel: w2126 -> [w2141 _]
                      frame True {
                        n1110 = stacked-sequence {
                          tunnel: w2144 -> [w2148 _]
                          tunnel: w2143 -> [w2146 w2152]
                          tunnel: w2142 -> [_ w2155]
                          tunnel: w2141 -> [w2145 _]
                          frame #0 {
                            n1111 = Build Array(w2146) -> (w2149:string[])
                            n1112 = Build Array(w2148) -> (w2147:dbl[])
                            n1113 = TDMS Write(0:w2145, 5:"TEST PASS", 7:w2149, 9:w2147) -> (15:w2151:errorcluster)  [unwired: 2 in, 3 out]
                            n1114 = local write "data file error"(w2151) -> ()
                          }
                          frame #1 {
                            n1115 = Bundle(cluster=w2155, "STATUS"=w2152) -> (w2153:T4)  [unwired: 2 in]
                            n1116 = local write "RESULT LAB01-2"(TRUE) -> ()
                            n1117 = local write "DISP LAB01-2"(w2153) -> ()
                          }
                        }
                      }
                      frame False {
                      }
                    }
                  }
                }
              }
              frame #2 {
                # "LAB02-1"
                n1118 = Less?(x=w2156, y=2) -> (x < y?=w2159:bool)
                n1119 = local read "DISP LAB02-1"() -> (w2161:T4)
                n1120 = Unbundle(w2161) -> ("STATUS"=w2162:string)  [unwired: 2 out]
                n1121 = Equal?(x=w2162, y="RUN") -> (x = y?=w2158:bool)
                n1122 = And(x=w2158, y=w2159) -> (x .and. y?=w2157:bool)
                n1123 = case shown="True" w2157 {
                  tunnel: w2161 -> [_ w2167]
                  tunnel: w2156 -> [_ w2171]
                  frame False {
                  }
                  frame True {
                    n1124 = local read "SET LAB02-1"() -> (w2173:T5)
                    n1125 = local read "TDMS LAB02-1"() -> (w2166:refnum<k34>)
                    n1126 = Unbundle(w2167) -> ("CYCLE"=w2172:dbl)  [unwired: 2 out]
                    n1127 = Unbundle(w2173) -> ("CYCLES"=w2164:dbl, "T-RISE mins"=w2170:dbl)  [unwired: 3 out]
                    n1128 = case shown="\"T-RISE TEST\"" w2171 {
                      tunnel: w2170 -> [_ _ w2180]
                      tunnel: [w2175 w2177 w2180] -> w2169
                      tunnel: w2164 -> [w2175 w2177 _]
                      tunnel: ["CHART PASS" "CYCLE PASS" "T-RISE PASS"] -> w2168
                      frame "CHART TEST", Default {
                      }
                      frame "CYCLE TEST" {
                      }
                      frame "T-RISE TEST" {
